vi "DTMF Packet Transmitter.vi"() -> ()   [LabVIEW 2011]
uses:
  <vilib>/addons/Modulation/Digital/General/MT Generate PSK System Parameters(M).vi
  <instrlib>/niUSRP/niUSRP Write Tx Data (CDB Cluster).vi
  <vilib>/addons/Modulation/niDMT.lvlib
panel:
  in  "autoscale":bool
  out "Constellation Graph":T1(graph)
  out "Symbol Rate\n[symbols/sec]":dbl=25000.0 format="%#.6p"
  in  "stop":bool
  in  "Tab Control":T2(tab)
  in  "Packet Parameters":T3={"Guard Bits "=30, "Sync Bits"=20, "Message Bits"=1024}
  in  "Packet Pad \n[samples]":i32=200
  in  "Blank Frame \n[samples]":i32=500
  out "Number of Packets in Message":i32=46
  in  "PN sequence order\nfor Sync Bits":i32=31 caption="PN sequence order (9)"
  in  "DTMF Settings":T4={"Phone Number"="", "Dial Tone"=FALSE, "Quantization Level"=4, "\nGray Encoding"=FALSE} {"Quantization Level" items=["2"=2, "4"=4, "8"=8, "16"=16]}
  out "Transmitted DTMF Signal":dbl[][](graph)
  in  "Select PSK Modulation Format":T5(tab)=enum."QPSK" caption="PSK"
  in  "BPSK System Parameters":T6={"Samples per Symbol"=8, "symbol map"=[], "Differential PSK"=enum."disable", "PSK type"=0} {"PSK type" items=["normal", "shifted", "offset"]; "symbol map" format="%.3f"}
  in  "QPSK System Parameters":T6={"Samples per Symbol"=8, "symbol map"=[], "Differential PSK"=enum."disable", "PSK type"=0} {"PSK type" items=["normal", "shifted", "offset"]; "symbol map" format="%.3f"}
  in  "pi/4 DQPSK System Parameters":T6={"Samples per Symbol"=8, "symbol map"=[], "Differential PSK"=enum."enable", "PSK type"=1} {"PSK type" items=["normal", "shifted", "offset"]; "symbol map" format="%.3f"}
  in  "OQPSK System Parameters":T6={"Samples per Symbol"=8, "symbol map"=[], "Differential PSK"=enum."disable", "PSK type"=2} {"PSK type" items=["normal", "shifted", "offset"]; "symbol map" format="%.3f"}
  in  "8-PSK System Parameters":T6={"Samples per Symbol"=8, "symbol map"=[], "Differential PSK"=enum."disable", "PSK type"=0} {"PSK type" items=["normal", "shifted", "offset"]; "symbol map" format="%.3f"}
  in  "16-PSK System Parameters":T6={"Samples per Symbol"=8, "symbol map"=[], "Differential PSK"=enum."disable", "PSK type"=0} {"PSK type" items=["normal", "shifted", "offset"]; "symbol map" format="%.3f"}
  in  "M":i32=4 min=2 step=2
  in  "Custom System Parameters":T6={"Samples per Symbol"=8, "symbol map"=[], "Differential PSK"=enum."disable", "PSK type"=0} {"PSK type" items=["normal", "shifted", "offset"]; "symbol map" format="%.3f"}
  in  "Pulse Shaping Filter Parameters":T7={"Alpha"=0.5, "Filter Length"=6, "TX Filter"=enum."Root Raised Cos"} caption="Pulse Shaping Filter" {"Alpha" format="%.2f"}
  in  "Tx Parameters":T8={"Tx IQ Sampling\nRate [s/sec]"=200000.0, "Tx Frequency [Hz]"=915000000.0, "Tx Gain [dB]"=0.0, "Tx Antenna"="TX1"} {"Tx Gain [dB]" format="%#.6p"; "Tx Frequency [Hz]" format="%#.6p"; "Tx IQ Sampling\nRate [s/sec]" format="%#.6p"}
  out "Actual Tx Parameters":T8={"Tx IQ Sampling\nRate [s/sec]"=200000.0, "Tx Frequency [Hz]"=2500000000.0, "Tx Gain [dB]"=0.0, "Tx Antenna"="TX1"} {"Tx Gain [dB]" format="%#.6p"; "Tx Frequency [Hz]" format="%#.6p"; "Tx IQ Sampling\nRate [s/sec]" format="%#.6p"}
  in  "USRP IP address":refnum<k15>="192.168.10.2"
  out "error out":errorcluster
  in  "Queue Length":i32=10
  # "DTMF Packet Transmitter"
  # "Guard\nBand"
  # "Sync\nSeq"
  # "Packet\nNumber"
  # "Pad\nData"
  # "Blank\nFrame"
  # "Data"
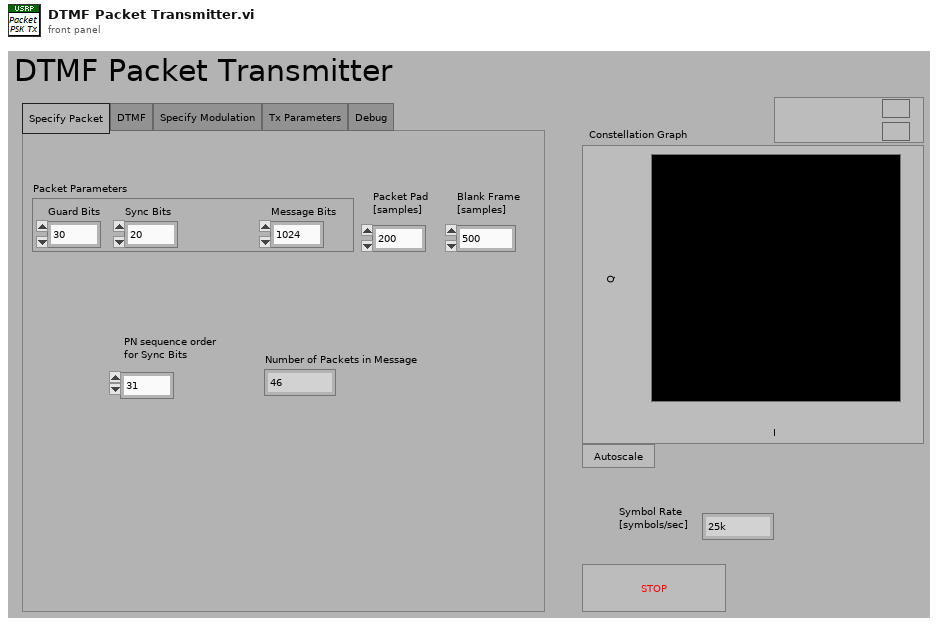
[diagram p1: front panel]
types:
  T1 = cluster{"Decimated Array":dbl[], "Decimated Array":dbl[]}[]
  T2 = enum32{"Specify Packet", "DTMF", "Specify Modulation", "Tx Parameters", "Debug"}
  T3 = cluster{"Guard Bits ":i32, "Sync Bits":i32, "Message Bits":i32}
  T4 = cluster{"Phone Number":string, "Dial Tone":bool, "Quantization Level":u16, "\nGray Encoding":bool}
  T5 = enum32{"BPSK", "QPSK", "pi/4DQPSK", "OQPSK", "8-PSK", "16-PSK", "Custom"}
  T6 = cluster{"Samples per Symbol":i32, "symbol map":cdb[], "Differential PSK":enum16{"disable", "enable"}, "PSK type":u16}
  T7 = cluster{"Alpha":dbl, "Filter Length":i32, "TX Filter":enum16{"none", "Raised Cosine", "Root Raised Cos", "Gaussian"}}
  T8 = cluster{"Tx IQ Sampling\nRate [s/sec]":dbl, "Tx Frequency [Hz]":dbl, "Tx Gain [dB]":dbl, "Tx Antenna":string}
  T9 = cluster{"samples per symbol (16)":i32, "symbol map":cdb[], "differential PSK":enum16{"disable", "enable"}, "PSK type":u16}
  T10 = cluster{"s? t:f":cluster{"t0":dbl, "dt":dbl, "Y":cdb[]}, i32}
  T11 = cluster{"output complex waveform":cluster{"t0":dbl, "dt":dbl, "Y":cdb[]}, i32}
  T12 = cluster{"constellation":dbl[], "oversampled data":dbl[]}[]
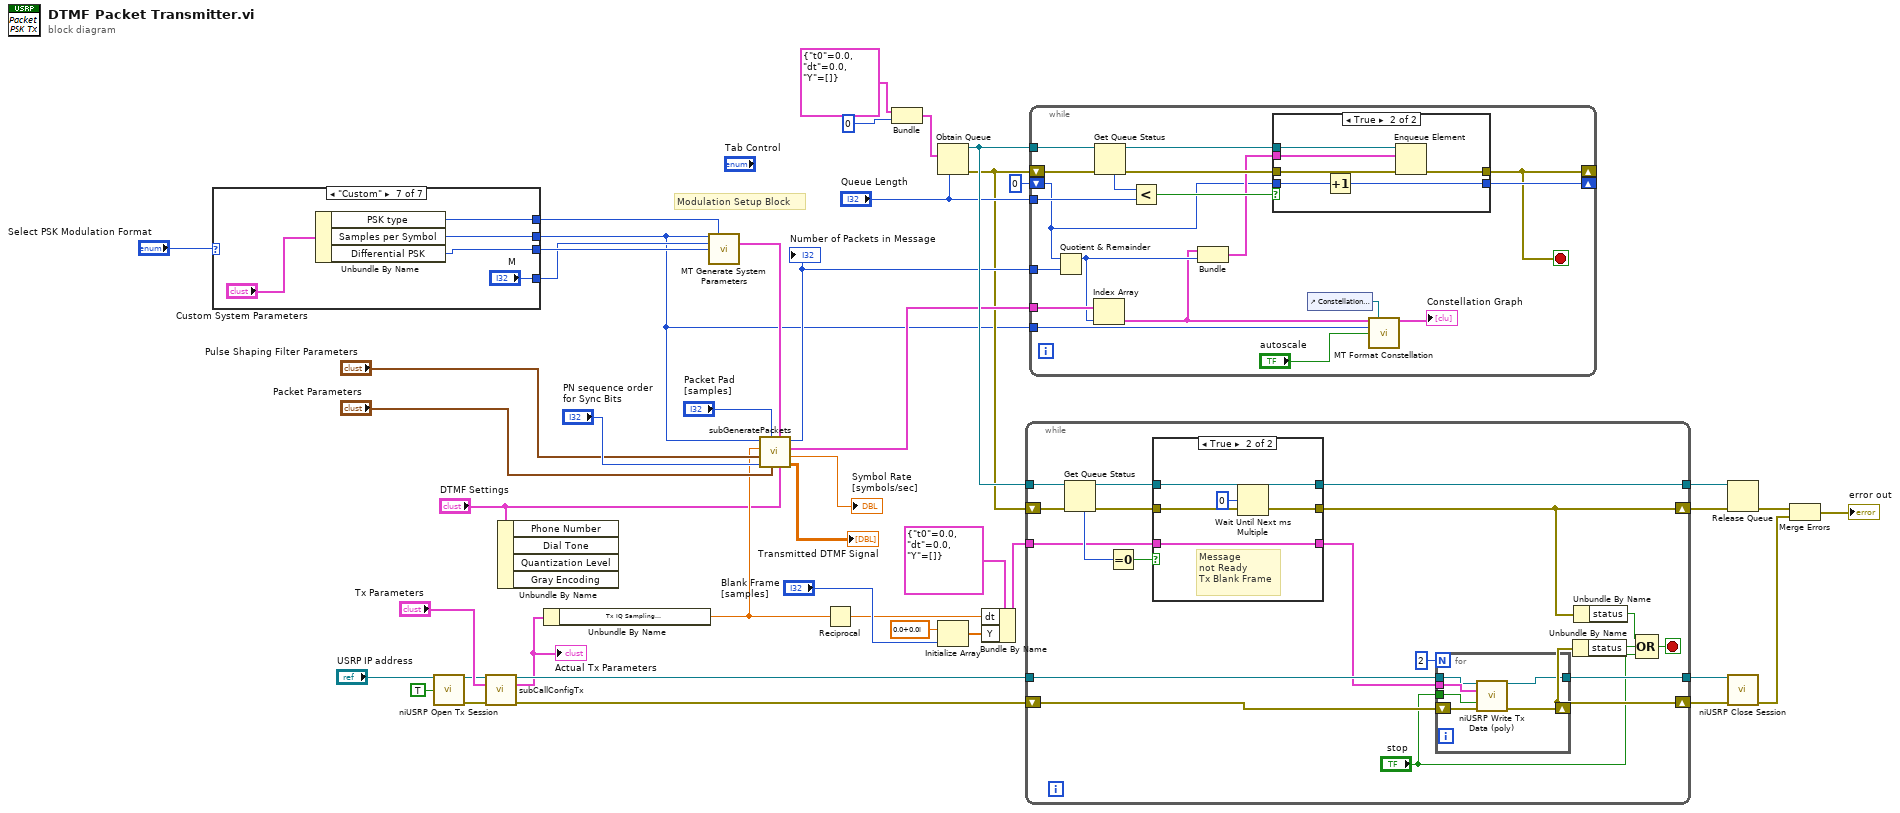
[diagram p0: block diagram]
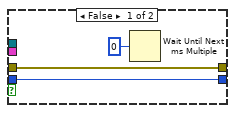
[diagram p2: hidden frame]
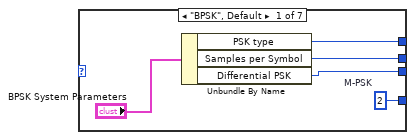
[diagram p3: hidden frame]
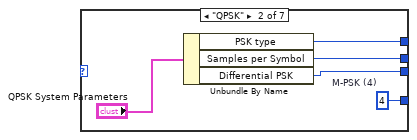
[diagram p4: hidden frame]
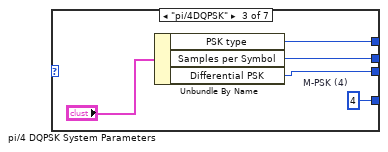
[diagram p5: hidden frame]
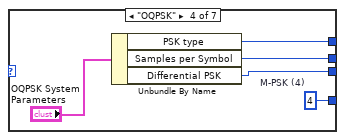
[diagram p6: hidden frame]
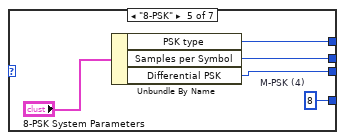
[diagram p7: hidden frame]
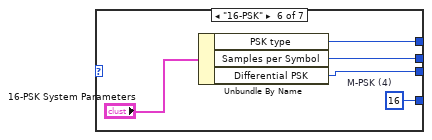
[diagram p8: hidden frame]
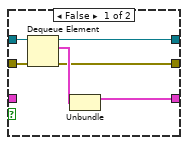
[diagram p9: hidden frame]
diagram:
  # "Modulation Setup Block"
  n1 = case shown="\"Custom\"" "Select PSK Modulation Format" {
    tunnel: [w46 w50 w58 w63 w68 w74 w77] -> w4
    tunnel: [w47 w52 w57 w62 w67 w73 w78] -> w43
    tunnel: [w49 w54 w59 w64 w66 w72 "M"] -> w25
    tunnel: [w48 w53 w56 w61 w69 w71 w79] -> w12
    frame "BPSK", Default {
      w49 = 2  # M-PSK
      n2 = Unbundle By Name("BPSK System Parameters") -> ("PSK type"=w48:u16, "Samples per Symbol"=w46:i32, "Differential PSK"=w47:enum16{"disable", "enable"})
    }
    frame "QPSK" {
      w54 = 4  # M-PSK (4)
      n3 = Unbundle By Name("QPSK System Parameters") -> ("PSK type"=w53:u16, "Samples per Symbol"=w50:i32, "Differential PSK"=w52:enum16{"disable", "enable"})
    }
    frame "pi/4DQPSK" {
      w59 = 4  # M-PSK (4)
      n4 = Unbundle By Name("pi/4 DQPSK System Parameters") -> ("PSK type"=w56:u16, "Samples per Symbol"=w58:i32, "Differential PSK"=w57:enum16{"disable", "enable"})
    }
    frame "OQPSK" {
      w64 = 4  # M-PSK (4)
      n5 = Unbundle By Name("OQPSK System Parameters") -> ("PSK type"=w61:u16, "Samples per Symbol"=w63:i32, "Differential PSK"=w62:enum16{"disable", "enable"})
    }
    frame "8-PSK" {
      w66 = 8  # M-PSK (4)
      n6 = Unbundle By Name("8-PSK System Parameters") -> ("PSK type"=w69:u16, "Samples per Symbol"=w68:i32, "Differential PSK"=w67:enum16{"disable", "enable"})
    }
    frame "16-PSK" {
      w72 = 16  # M-PSK (4)
      n7 = Unbundle By Name("16-PSK System Parameters") -> ("PSK type"=w71:u16, "Samples per Symbol"=w74:i32, "Differential PSK"=w73:enum16{"disable", "enable"})
    }
    frame "Custom" {
      n8 = Unbundle By Name("Custom System Parameters") -> ("PSK type"=w79:u16, "Samples per Symbol"=w77:i32, "Differential PSK"=w78:enum16{"disable", "enable"})
    }
  }
  n9 = call <instrlib>:"niUSRP Open Tx Session.vi"("device names"="USRP IP address", "reset"=TRUE) -> ("session handle out"=w16:refnum<k15>, "error out"=w15:errorcluster)  [unwired: 12 in]
  n10 = call "subCallConfigTx.vi"("session handle"=w16, "Tx Parameters"="Tx Parameters", "error in"=w15) -> ("session handle out"=w24:refnum<k15>, "Actual Tx Parameters"=w23:T8, "error out"=w29:errorcluster)  [unwired: 10 in]
  "Actual Tx Parameters" <- w23
  n11 = Unbundle By Name("DTMF Settings") -> ()  [unwired: 4 out]
  n12 = Unbundle By Name(w23) -> ("Tx IQ Sampling\nRate [s/sec]"=w5:dbl)
  n13 = call-poly <vilib>:"MT Generate System Parameters.vi"("samples per symbol (16)"=w4, "PSK type"=w12, "M-PSK (4)"=w25, "differential PSK"=w43) -> ("PSK system parameters"=w13:T9)  [unwired: 9 in, 2 out]
  n14 = call "subGeneratePackets.vi"("DTMF Settings"="DTMF Settings", "PSK system parameters"=w13, "Packet Parameters"="Packet Parameters", "Packet Pad \n[samples]"="Packet Pad \n[samples]", "PN sequence order\nfor Sync Bits"="PN sequence order\nfor Sync Bits", "Pulse Shaping Filter Parameters"="Pulse Shaping Filter Parameters", "Tx IQ Sampling\nRate [s/sec]"=w5, "Samples per Symbol"=w4) -> ("TX DTMF Signal"=→"Transmitted DTMF Signal":dbl[][], "Symbol Rate"=→"Symbol Rate\n[symbols/sec]":dbl, "Packets"=w31:cluster{"t0":dbl, "dt":dbl, "Y":cdb[]}[], "Number of Packets"=w22:i32)
  "Number of Packets in Message" <- w22
  n15 = Reciprocal(x=w5) -> (1/x=w26:dbl)
  n16 = Bundle("s? t:f"=cluster{"t0":dbl, "dt":dbl, "Y":cdb[]} {"t0"=0.0, "dt"=0.0, "Y"=[]}, 0) -> (w34:T10)  [unwired: 1 in]
  n17 = Obtain Queue(max queue size (-1, unlimited)="Queue Length", element data type=w34) -> (queue out=w40:refnum<queue>, error out=w18:errorcluster)  [unwired: 3 in, 1 out]
  n18 = Initialize Array(cdb 0.0+0.0i ("element"), "Blank Frame \n[samples]") -> (w39:cdb[])
  n19 = Bundle By Name(cluster=cluster{"t0":dbl, "dt":dbl, "Y":cdb[]} {"t0"=0.0, "dt"=0.0, "Y"=[]} ("s? t:f"), "dt"=w26, "Y"=w39) -> (w38:cluster{"t0":dbl, "dt":dbl, "Y":cdb[]})
  n20 = while {
    tunnel: w24 -> [w89]
    shift-right: [w86] -> w28
    shift-left: w29 -> [w90]
    tunnel: w40 -> [w98]
    tunnel: w38 -> [w95]
    tunnel: [w94] -> w37
    tunnel: [w88] -> w27
    shift-right: [w82] -> w36
    shift-left: w18 -> [w91]
    stop <- w85 stop-if-true
    n21 = Get Queue Status(queue=w98, error in (no error)=w91) -> (queue out=w93:refnum<queue>, error out=w92:errorcluster, # elements in queue=w97:i32)  [unwired: 1 in, 5 out]
    n22 = Equal To 0?(x=w97) -> (x = 0?=w96:bool)
    n23 = case shown="True" w96 {
      tunnel: w95 -> [_ w114]
      tunnel: [w106 w114] -> w80
      tunnel: [w110 w112] -> w94
      tunnel: [w105 w113] -> w82
      tunnel: w93 -> [w109 w112]
      tunnel: w92 -> [w108 w113]
      frame False {
        n24 = Dequeue Element(queue=w109, error in (no error)=w108) -> (queue out=w110:refnum<queue>, element=w107:T10, error out=w105:errorcluster)  [unwired: 1 in, 1 out]
        n25 = Unbundle(w107) -> ("s? t:f"=w106:cluster{"t0":dbl, "dt":dbl, "Y":cdb[]})  [unwired: 1 out]
      }
      frame True {
        # "Message\nnot Ready\nTx Blank Frame"
        n26 = Wait Until Next ms Multiple(millisecond multiple=u32 0) -> ()  [unwired: 1 out]
      }
    }
    n27 = for {
      N: 2 -> [_]
      tunnel: w80 -> [w103]
      tunnel: w89 -> [w102]
      tunnel: [w101] -> w88
      tunnel: "stop" -> [w100]
      shift-right: [w99] -> w86
      shift-left: w90 -> [w104]
      n28 = call-poly <instrlib>:"niUSRP Write Tx Data (poly).vi"("session handle"=w102, "data"=w103, "end of data?"=w100, "error in (no error)"=w104) -> ("session handle out"=w101:refnum<k15>, "error out"=w99:errorcluster)  [unwired: 10 in]
    }
    n29 = Unbundle By Name(w86) -> ("status"=w87:bool)
    n30 = Unbundle By Name(w82) -> ("status"=w81:bool)
    n31 = Compound Arithmetic op=OR(w81, w87, "stop") -> (w85:bool)
  }
  n32 = while {
    tunnel: w40 -> [w133]
    shift-right: [w126] -> _
    shift-left: 0 -> [w122]
    tunnel: w31 -> [w123]
    tunnel: "Queue Length" -> [w125]
    tunnel: w22 -> [w124]
    shift-right: [w120] -> _
    shift-left: w18 -> [w128]
    tunnel: w4 -> [w117]
    stop <- w120 stop-if-true
    n33 = Quotient & Remainder(x=w122, y=w124) -> (x-y*floor(x/y)=w121:i32)  [unwired: 1 out]
    n34 = Index Array(array=w123, index=w121) -> (element=w115:cluster{"t0":dbl, "dt":dbl, "Y":cdb[]})
    n35 = Get Queue Status(queue=w133, error in (no error)=w128) -> (queue out=w132:refnum<queue>, error out=w129:errorcluster, # elements in queue=w131:i32)  [unwired: 1 in, 5 out]
    n36 = Less?(x=w131, y=w125) -> (x < y?=w130:bool)
    n37 = Bundle("output complex waveform"=w115, w121) -> (w127:T11)  [unwired: 1 in]
    n38 = case shown="True" w130 {
      tunnel: w129 -> [w134 w142]
      tunnel: w132 -> [_ w141]
      tunnel: [w134 w140] -> w120
      tunnel: w127 -> [_ w139]
      tunnel: w122 -> [w136 w138]
      tunnel: [w136 w137] -> w126
      frame False {
        n39 = Wait Until Next ms Multiple(millisecond multiple=u32 0) -> ()  [unwired: 1 out]
      }
      frame True {
        n40 = Increment(x=w138) -> (x+1=w137:i32)
        n41 = Enqueue Element(queue=w141, element=w139, error in (no error)=w142) -> (error out=w140:errorcluster)  [unwired: 1 in, 2 out]
      }
    }
    n42 = control-ref of="Constellation Graph"() -> (w118:refnum<vi>)
    n43 = call <vilib>:"MT Format Constellation.vi"("waveform"=w115, "constellation reference"=w118, "samples per symbol"=w117, "autoscale"="autoscale") -> ("constellation graph"=→"Constellation Graph":T12)  [unwired: 1 in, 10 out]
  }
  n44 = Release Queue(queue=w37, error in (no error)=w36) -> (error out=w11:errorcluster)  [unwired: 3 out]
  n45 = call <instrlib>:"niUSRP Close Session.vi"("session handle"=w27, "error in (no error)"=w28) -> ("error out"=w10:errorcluster)  [unwired: 13 in]
  n46 = Merge Errors(w11, w10) -> (→"error out":errorcluster)
